vi "Add Noise.vi"(6 "Sampling":T1, 8 "error in (no error)":errorcluster, 11 "AI []":waveform(dbl)[](array[waveform])) -> (0 "error out":errorcluster, 3 "AI + Noise":waveform(dbl)[](array[waveform]))   [LabVIEW 2019, in "Instrument.DAQ.lvclass"]
uses:
  Instrument.DAQ.lvclass
  <vilib>/Analysis/NI_AALPro.lvlib
  <vilib>/Analysis/2dsp.llb/Real FFT.vi
  <vilib>/Analysis/2dsp.llb/Inverse Real FFT.vi
  <vilib>/measure/NI_MABase.lvlib
  Typedefs/DAQ.Sampling.Sampling--Cluster.ctl
panel:
  in  "Noise Cluster":T2={"1/f vs. Uniform "=1.0, "60Hz Amplitude"=0.005, "Gauss/Unif %"=0.5, "Noise Amp"=0.005}
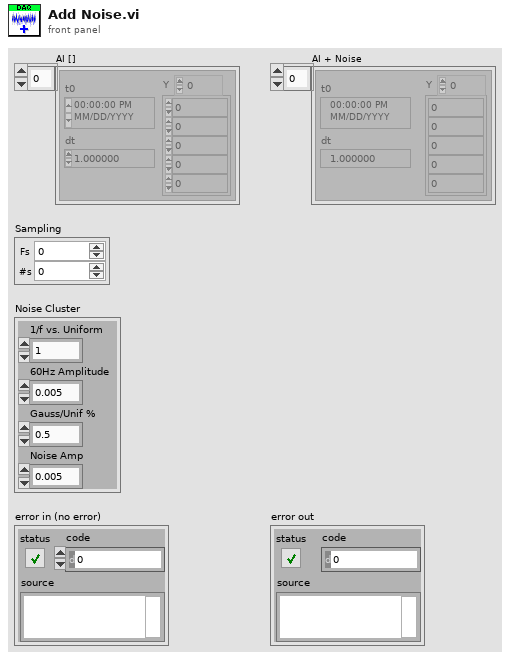
[diagram p1: front panel]
types:
  T1 = typedef "Instrument.DAQ.lvclass/DAQ.Sampling.Sampling--Cluster.ctl" = cluster{"Fs":dbl, "#s":i32}
  T2 = cluster{"1/f vs. Uniform ":dbl, "60Hz Amplitude":dbl, "Gauss/Unif %":dbl, "Noise Amp":dbl}
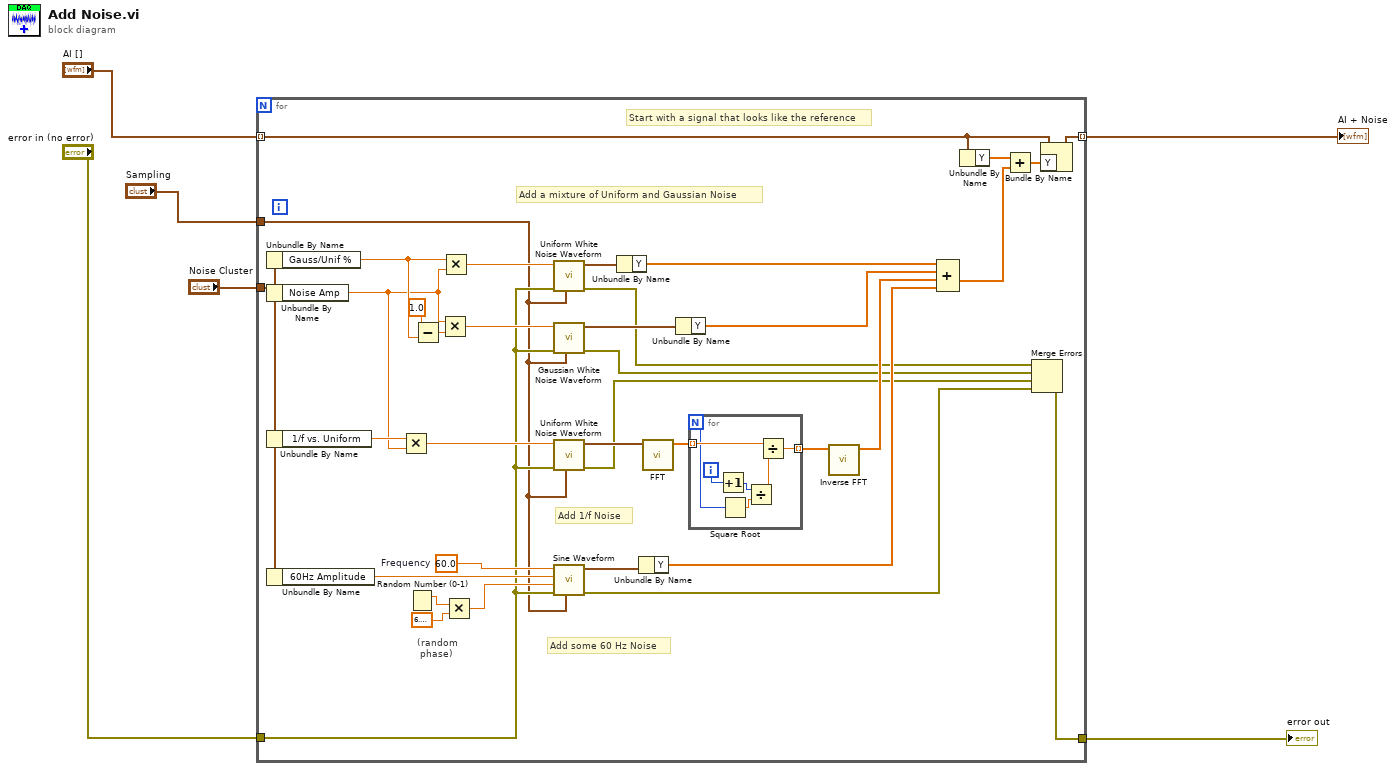
[diagram p0: block diagram]
diagram:
  n1 = for {
    tunnel: "Noise Cluster" -> [w22]
    tunnel: "Sampling" -> [w12]
    tunnel: [w13] -> w6 mode=indexing
    tunnel: "error in (no error)" -> [w16]
    tunnel: [w7] -> w2
    tunnel: "AI []" -> [w8] mode=indexing
    w17 = 60.0  # Frequency
    # "Start with a signal that looks like the reference"
    # "Add 1/f Noise"
    # "(random\n phase)"
    # "Add some 60 Hz Noise"
    # "Add a mixture of Uniform and Gaussian Noise"
    n2 = Unbundle By Name(w22) -> ("Gauss/Unif %"=w27:dbl)
    n3 = Unbundle By Name(w22) -> ("Noise Amp"=w9:dbl)
    n4 = Unbundle By Name(w22) -> ("1/f vs. Uniform"=w26:dbl)
    n5 = Unbundle By Name(w22) -> ("60Hz Amplitude"=w25:dbl)
    n6 = Multiply(x=w26, y=w9) -> (x*y=w33:dbl)
    n7 = Random Number (0-1)() -> (number: 0 to 1=w37:dbl)
    n8 = Subtract(x=1.0, y=w27) -> (x-y=w40:dbl)
    n9 = Multiply(x=w9, y=w40) -> (x*y=w21:dbl)
    n10 = Multiply(x=w27, y=w9) -> (x*y=w20:dbl)
    n11 = Multiply(x=w37, y=6.283185307179586) -> (x*y=w19:dbl)
    n12 = call <vilib>:"Uniform White Noise Waveform.vi"("sampling info"=w12, "error in (no error)"=w16, "amplitude"=w20) -> ("error out"=w10:errorcluster, "signal out"=w41:waveform(dbl))  [unwired: 7 in]
    n13 = call <vilib>:"Gaussian White Noise Waveform.vi"("sampling info"=w12, "error in (no error)"=w16, "standard deviation"=w21) -> ("error out"=w11:errorcluster, "signal out"=w42:waveform(dbl))  [unwired: 7 in]
    n14 = call <vilib>:"Uniform White Noise Waveform.vi"("sampling info"=w12, "error in (no error)"=w16, "amplitude"=w33) -> ("error out"=w15:errorcluster, "signal out"=w32:waveform(dbl))  [unwired: 7 in]
    n15 = call <vilib>:"Sine Waveform.vi"("sampling info"=w12, "error in (no error)"=w16, "phase"=w19, "amplitude"=w25, "frequency"=w17) -> ("error out"=w14:errorcluster, "signal out"=w36:waveform(dbl))  [unwired: 5 in]
    n16 = Unbundle By Name(w41) -> ("Y"=w35:dbl[])
    n17 = Unbundle By Name(w36) -> ("Y"=w31:dbl[])
    n18 = call-poly <vilib>:"FFT.vi"("X"=w32) -> ("FFT {X}"=w18:cdb[])  [unwired: 9 in, 1 out]
    n19 = Unbundle By Name(w42) -> ("Y"=w28:dbl[])
    n20 = for {
      N -> [w46]
      tunnel: [w49] -> w34 mode=indexing
      tunnel: w18 -> [w48] mode=indexing
      i -> [w47]
      n21 = Increment(x=w47) -> (x+1=w44:i32)
      n22 = Square Root(x=w46) -> (sqrt(x)=w45:dbl)
      n23 = Divide(x=w44, y=w45) -> (x/y=w43:dbl)
      n24 = Divide(x=w48, y=w43) -> (x/y=w49:cdb)
    }
    n25 = call-poly <vilib>:"Inverse FFT.vi"("FFT {X}"=w34) -> ("X"=w30:dbl[])  [unwired: 9 in, 1 out]
    n26 = Compound Arithmetic op=ADD(w35, w28, w30, w31) -> (w29:dbl[])
    n27 = Unbundle By Name(w8) -> ("Y"=w24:dbl[])
    n28 = Add(x=w24, y=w29) -> (x+y=w23:dbl[])
    n29 = Merge Errors(w10, w11, w15, w14) -> (w7:errorcluster)
    n30 = Bundle By Name(cluster=w8, "Y"=w23) -> (w13:waveform(dbl))
  }
  "AI + Noise" <- w6
  "error out" <- w2
